vi "Generate New File.vi"(8 "error in":errorcluster, 11 "File Obs in":refnum<class "File Observer.lvclass">) -> (0 "error out":errorcluster, 2 "File Ref Out":refnum<file>, 3 "File Obs out":refnum<class "File Observer.lvclass">)   [LabVIEW 2014, in "File Observer.lvclass"]
doc: "Generate a New File for use by the observer based on the caller defined File Name and Data Path. If there is a file open, close it."
uses:
  File Observer.lvclass
  File Observer.lvclass/File Observer.ctl
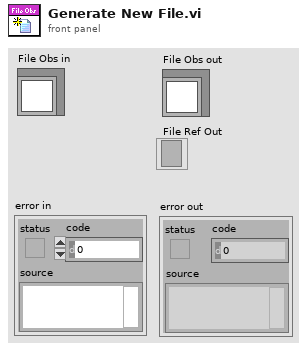
[diagram p1: front panel]
types:
  T1 = enum16{"open", "replace", "create", "open or create", "replace or create", "replace or create with confirmation"}
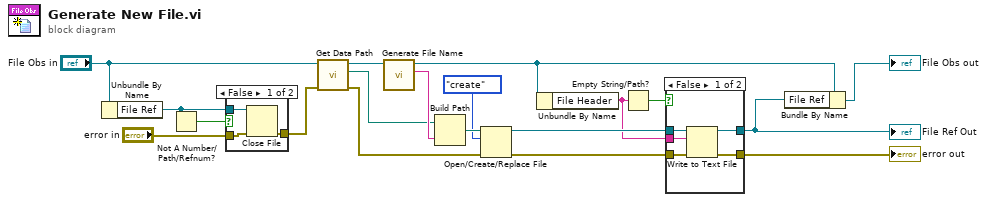
[diagram p0: block diagram]
diagram:
  n1 = Unbundle By Name("File Obs in") -> ("File Ref"=w10:refnum<file>)
  n2 = Not A Number/Path/Refnum?(number/path/refnum=w10) -> (NaN/Path/Refnum?=w11:bool)
  n3 = case shown="False" w11 {
    tunnel: w10 -> [w22 _]
    tunnel: "error in" -> [w21 w23]
    tunnel: [w20 w23] -> w8
    frame False {
      n4 = Close File(refnum=w22, error in=w21) -> (error out=w20:errorcluster)  [unwired: 1 out]
    }
    frame True {
    }
  }
  n5 = call-dynamic "Get Data Path.vi"("error in"=w8, "File Observer in"="File Obs in") -> ("error out"=w16:errorcluster, "path out"=w13:path, "File Observer out"=w14:refnum<class "File Observer.lvclass">)  [unwired: 7 in]
  n6 = call-dynamic "Generate File Name.vi"("File Obs in"=w14) -> ("File Name"=w15:string, "File Obs out"=w7:refnum<class "File Observer.lvclass">)  [unwired: 9 in]
  n7 = Build Path(base path=w13, name or relative path=w15) -> (appended path=w18:path)
  n8 = Open/Create/Replace File(file path (use dialog)=w18, error in=w16, operation (0:open)=T1."create") -> (refnum out=w6:refnum<file>, error out=w5:errorcluster)  [unwired: 4 out]
  n9 = Unbundle By Name(w7) -> ("File Header"=w1:string)
  n10 = Empty String/Path?(string/path=w1) -> (empty?=w2:bool)
  n11 = case shown="False" w2 {
    tunnel: w6 -> [w28 w30]
    tunnel: w5 -> [w27 w29]
    tunnel: [w26 w30] -> w4
    tunnel: [w25 w29] -> w3
    tunnel: w1 -> [w24 _]
    frame False {
      n12 = Write to Text File(file (use dialog)=w28, text=w24, error in=w27) -> (refnum out=w26:refnum<file>, error out=w25:errorcluster)  [unwired: 1 in, 1 out]
    }
    frame True {
    }
  }
  "error out" <- w3
  "File Ref Out" <- w4
  n13 = Bundle By Name(cluster=w7, "File Ref"=w4) -> (→"File Obs out":refnum<class "File Observer.lvclass">)
